vi "PMS7003_init_subVin.vi"(8 "error in":errorcluster, 10 "Init":bool, 11 "VISA Refnum in":refnum<visa-resource-name>) -> (0 "error out":errorcluster, 3 "VISA Refnum out":refnum<visa-resource-name>)   [LabVIEW 2019]
doc: "Initialize PMS7003 sensor with one shot mode if init bool == true or ask for data if init bool == false \nFor PMS7003 :\nBaud rate: 9600\nData bits: 8\nParinty: none\nStop bits: 1\nFslow control none"
uses:
  <vilib>/Instr/_visa.llb/VISA Configure Serial Port (Instr).vi
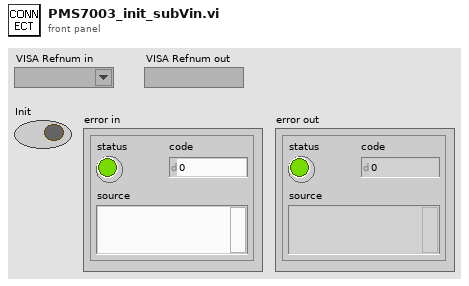
[diagram p1: front panel]
types:
  T1 = cluster{"baud rate":u32, "data bits":u16, "parity":enum16{"None", "Odd", "Even", "Mark", "Space"}, "stop bits":u16, "flow control":u16}
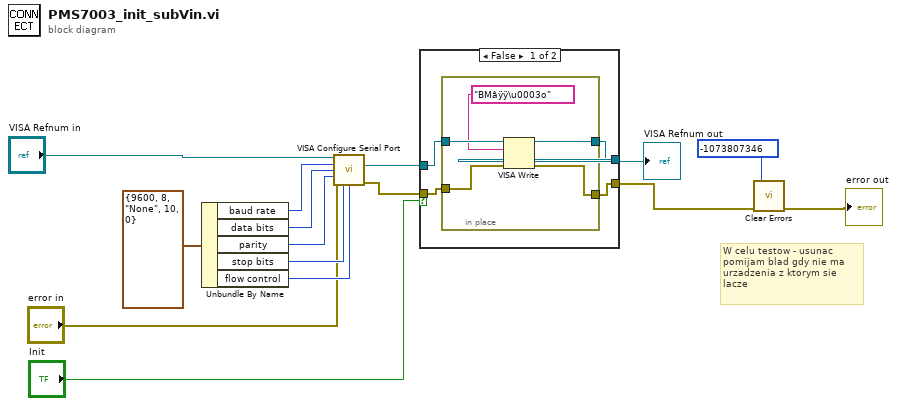
[diagram p0: block diagram]
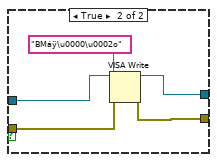
[diagram p2: hidden frame]
diagram:
  # "W celu testow - usunac \npomijam blad gdy nie ma \nurzadzenia z ktorym sie \nlacze"
  n1 = Unbundle By Name(T1 {"baud rate"=9600, "data bits"=8, "parity"=enum."None", "stop bits"=10, "flow control"=0} ("input cluster")) -> ("baud rate"=w9:u32, "data bits"=w8:u16, "parity"=w7:enum16{"None", "Odd", "Even", "Mark", "Space"}, "stop bits"=w6:u16, "flow control"=w10:u16)
  n2 = call-poly "VISA Configure Serial Port"("VISA resource name"="VISA Refnum in", "baud rate (9600)"=w9, "data bits (8)"=w8, "parity (0:none)"=w7, "error in (no error)"="error in", "stop bits (10: 1 bit)"=w6, "flow control (0:none)"=w10) -> ("VISA resource name out"=w11:refnum<visa-resource-name>, "error out"=w12:errorcluster)  [unwired: 3 in, 4 out]
  n3 = case shown="False" "Init" {
    tunnel: w11 -> [w19 w27]
    tunnel: [w16 w29] -> w13
    tunnel: [w17 w28] -> w2
    tunnel: w12 -> [w18 w26]
    frame False {
      n4 = in-place {
        in-place-border: w19 -> [w24]
        in-place-border: w18 -> [w23]
        in-place-border: [w22] -> w17
        in-place-border: [w21] -> w16
        n5 = VISA Write(VISA resource name=w24, write buffer="BMâÿÿ\u0003o", error in (no error)=w23) -> (VISA resource name out=w21:refnum<visa-resource-name>, error out=w22:errorcluster)  [unwired: 1 out]
      }
    }
    frame True {
      n6 = VISA Write(VISA resource name=w27, write buffer="BMáÿ\u0000\u0002o", error in (no error)=w26) -> (VISA resource name out=w29:refnum<visa-resource-name>, error out=w28:errorcluster)  [unwired: 1 out]
    }
  }
  "VISA Refnum out" <- w13
  n7 = call <vilib>:"Clear Errors.vi"("error in (no error)"=w2, "specific error code to clear (0: all)"=-1073807346 ("y")) -> ("error out"=→"error out":errorcluster)  [unwired: 4 in, 1 out]
